vi "Excersie_6.vi"() -> ()   [LabVIEW 2013]
panel:
  in  "stop":bool
  out "error out":errorcluster
  in  "error in (no error)":errorcluster
  out "Square Root Value":dbl
  in  "Numeric":dbl
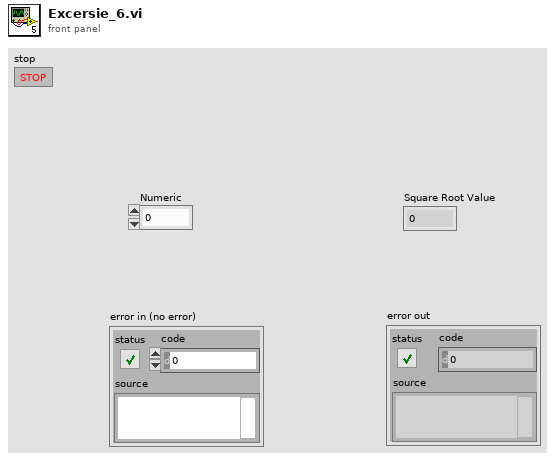
[diagram p1: front panel]
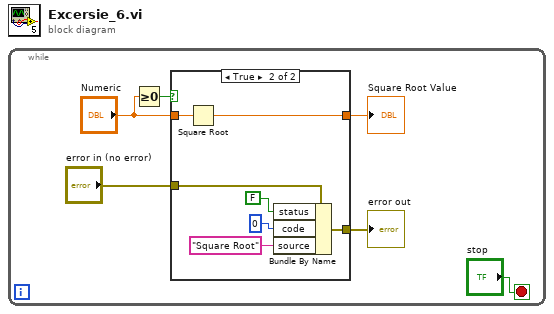
[diagram p0: block diagram]
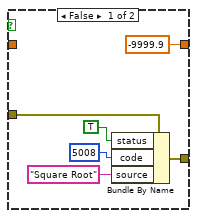
[diagram p2: hidden frame]
diagram:
  n1 = while {
    stop <- "stop" stop-if-true
    n2 = Greater Or Equal To 0?(x="Numeric") -> (x >= 0?=w6:bool)
    n3 = case shown="True" w6 {
      tunnel: "error in (no error)" -> [w10 w19]
      tunnel: "Numeric" -> [_ w14]
      tunnel: [-9999.9 w13] -> w4
      tunnel: [w11 w18] -> w2
      frame False {
        n4 = Bundle By Name(cluster=w10, "status"=TRUE, "code"=5008, "source"="Square Root") -> (w11:errorcluster)
      }
      frame True {
        n5 = Square Root(x=w14) -> (sqrt(x)=w13:dbl)
        n6 = Bundle By Name(cluster=w19, "status"=FALSE, "code"=0, "source"="Square Root") -> (w18:errorcluster)
      }
    }
    "Square Root Value" <- w4
    "error out" <- w2
  }
